vi "Reentrant Method.vi"(8 "error in (no error)":errorcluster, 10 "Numeric":dbl, 11 "Test Interface Mock in":refnum<class "Test Interface Mock.lvclass">) -> (0 "error out":errorcluster, 3 "Test Interface Mock out":refnum<class "Test Interface Mock.lvclass">)   [LabVIEW 2020, in "Test Interface Mock.lvclass"]
uses:
  Test Interface Mock.lvclass
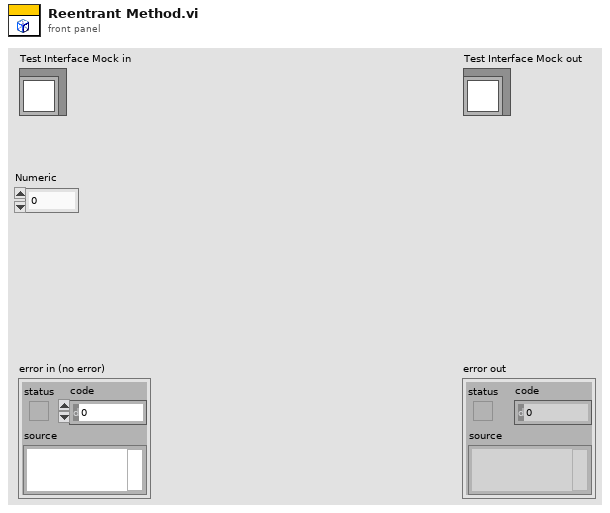
[diagram p1: front panel]
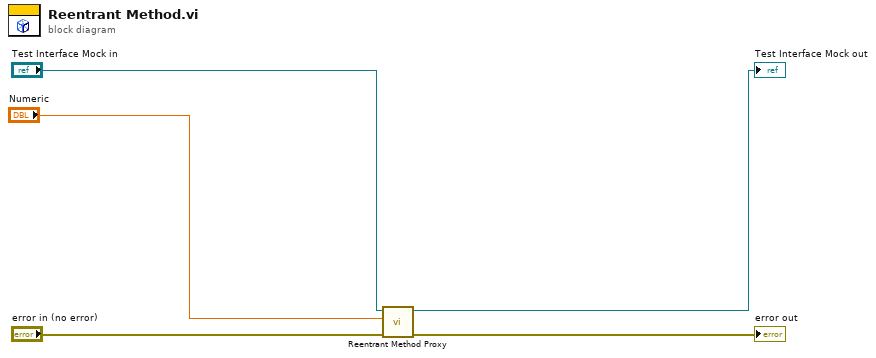
[diagram p0: block diagram]
diagram:
  n1 = call "Reentrant Method Proxy.vi"("error in (no error)"="error in (no error)", "Numeric in"="Numeric", "Test Interface Mock in"="Test Interface Mock in") -> ("error out"=→"error out":errorcluster, "Test Interface Mock out"=→"Test Interface Mock out":refnum<class "Test Interface Mock.lvclass">)  [unwired: 7 in]
